vi "1-2.vi"() -> ()   [LabVIEW 2018]
panel:
  out "X!":dbl
  out "∑X!":dbl
  in  "X":dbl
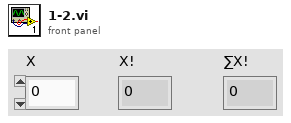
[diagram p1: front panel]
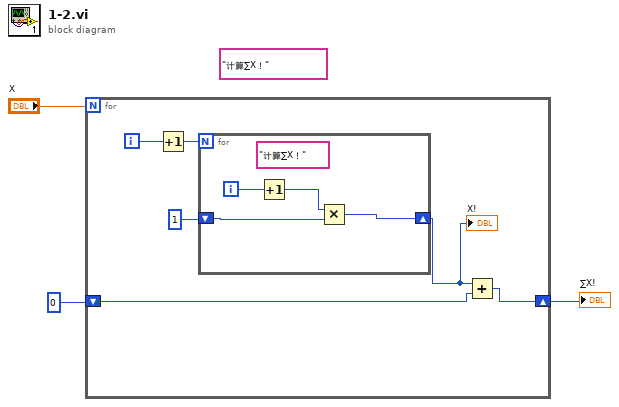
[diagram p0: block diagram]
diagram:
  (unwired) "计算∑X！"
  n1 = for {
    N: "X" -> [_]
    shift-right: [w5] -> w1
    shift-left: 0 -> [w6]
    i -> [w9]
    n2 = Increment(x=w9) -> (x+1=w7:i32)
    n3 = for {
      N: w7 -> [_]
      shift-right: [w10] -> w4
      shift-left: 1 -> [w11]
      i -> [w13]
      (unwired) "计算∑X！"
      n4 = Increment(x=w13) -> (x+1=w12:i32)
      n5 = Multiply(x=w12, y=w11) -> (x*y=w10:i32)
    }
    "X!" <- w4
    n6 = Add(x=w4, y=w6) -> (x+y=w5:i32)
  }
  "∑X!" <- w1
